vi "DAQmx Start Task.vi"(0 "task/channels in":refnum<k21>, 11 "error in":errorcluster) -> (4 "task out":refnum<k21>, 15 "error out":errorcluster)   [LabVIEW 2017]
doc: "Transitions the task to the running state to begin the measurement or generation. Using this VI is required for some applications and is optional for others."
uses:
  nilvaiu.dll
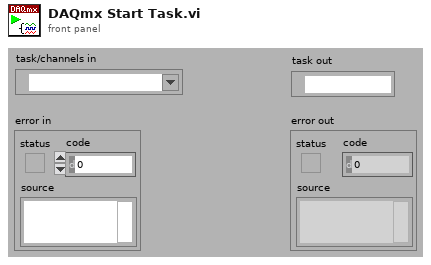
[diagram p1: front panel]
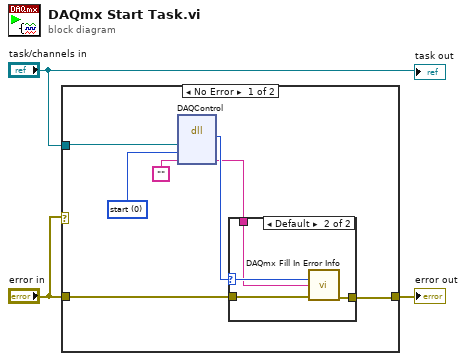
[diagram p0: block diagram]
diagram:
  n1 = case shown="No Error" "error in" {
    tunnel: [w5 w16] -> w3
    tunnel: "error in" -> [w6 w16]
    tunnel: "task/channels in" -> [w7 _]
    frame No Error {
      w4 = u16 0 items=["start"]
      n2 = dll-call lib="nilvaiu.*" fn="DAQControl"("taskID"=w7, "mode"=w4, "extendedErrorInfo"="") -> (w10:i32, "extendedErrorInfo"=w9:string)  [unwired: 3 in, 4 out]
      n3 = case shown="Default" w10 {
        selector: w10 -> [_ w14]
        tunnel: [w11 w15] -> w5
        tunnel: w9 -> [_ w13]
        tunnel: w6 -> [w11 w12]
        frame 0 {
        }
        frame Default {
          n4 = call "DAQmx Fill In Error Info.vi"("status code"=w14, "extended error info"=w13, "error in"=w12) -> ("error out"=w15:errorcluster)  [unwired: 1 in, 11 out]
        }
      }
    }
    frame Error {
    }
  }
  "error out" <- w3
  "task out" <- "task/channels in"
